vi "ball_demo.vi"() -> ()   [LabVIEW 2011]
panel:
  in  "stop":bool
  in  "Initial velocity":dbl(knob) scale=-15.0..15.0
  in  "Coefficient of Restitution":dbl(knob)=1.0 scale=0.0..1.5
  in  "Initial height":dbl(knob)=5.0 scale=5.0..20.0
  out "LabVIEW":cluster{dbl[], dbl[]}[](graph)
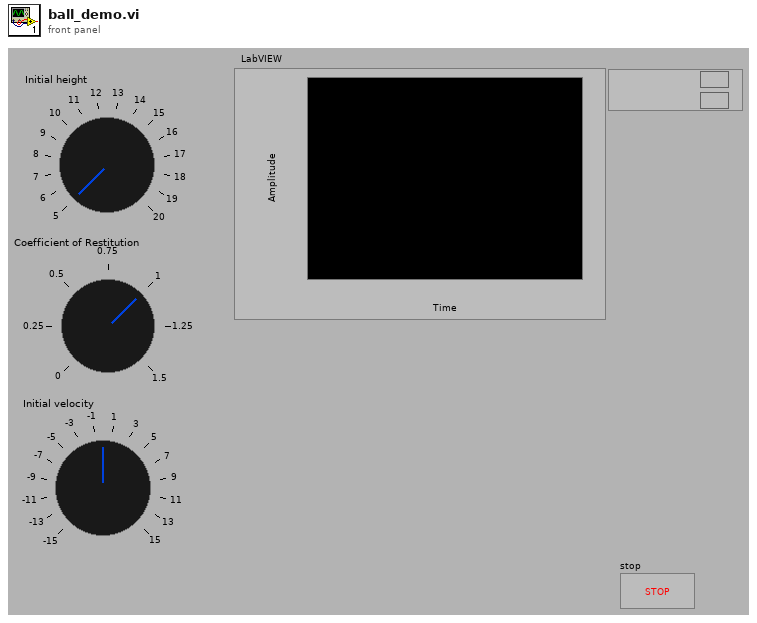
[diagram p1: front panel]
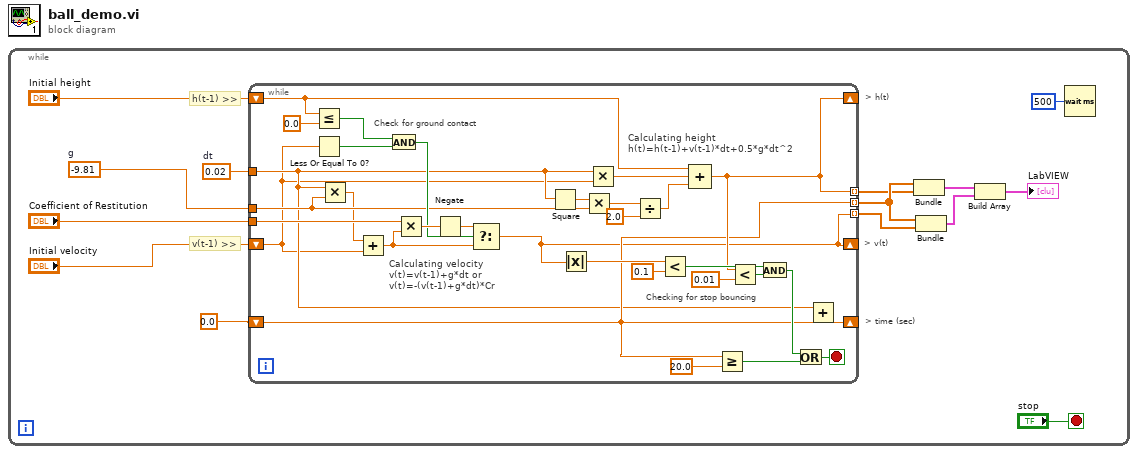
[diagram p0: block diagram]
diagram:
  n1 = while {
    stop <- "stop" stop-if-true
    w1 = 0.02  # dt
    w2 = -9.81  # g
    # "> v(t)"
    # "v(t-1) >>"
    # "h(t-1) >>"
    # "> h(t)"
    # "> time (sec)"
    n2 = while {
      tunnel: w1 -> [w19]
      tunnel: w2 -> [w27]
      shift-right: [w18] -> _
      shift-left: "Initial velocity" -> [w17]
      shift-right: [w23] -> _
      shift-left: "Initial height" -> [w38]
      tunnel: "Coefficient of Restitution" -> [w29]
      shift-right: [w21] -> _
      shift-left: 0.0 ("time") -> [w20]
      tunnel: [w23] -> w13 mode=indexing
      tunnel: [w18] -> w12 mode=indexing
      tunnel: [w20] -> w14 mode=indexing
      stop <- w34 stop-if-true
      # "Checking for stop bouncing"
      # "Calculating velocity\nv(t)=v(t-1)+g*dt or\nv(t)=-(v(t-1)+g*dt)*Cr"
      # "Check for ground contact"
      # "Calculating height\nh(t)=h(t-1)+v(t-1)*dt+0.5*g*dt^2"
      n3 = Less Or Equal?(x=w38, y=0.0) -> (x <= y?=w41:bool)
      n4 = Less Or Equal To 0?(x=w17) -> (x <= 0?=w40:bool)
      n5 = Multiply(x=w19, y=w27) -> (x*y=w16:dbl)
      n6 = Add(x=w16, y=w17) -> (x+y=w15:dbl)
      n7 = And(x=w41, y=w40) -> (x .and. y?=w39:bool)
      n8 = Multiply(x=w29, y=w15) -> (x*y=w43:dbl)
      n9 = Negate(x=w43) -> (-x=w42:dbl)
      n10 = Select(t=w42, s=w39, f=w15) -> (s? t:f=w18:dbl)
      n11 = Square(x=w19) -> (x^2=w28:dbl)
      n12 = Absolute Value(x=w18) -> (abs(x)=w36:dbl)
      n13 = Multiply(x=w28, y=w27) -> (x*y=w26:dbl)
      n14 = Multiply(x=w19, y=w17) -> (x*y=w45:dbl)
      n15 = Divide(x=w26, y=2.0) -> (x/y=w24:dbl)
      n16 = Less?(x=w36, y=0.1) -> (x < y?=w30:bool)
      n17 = Compound Arithmetic op=ADD(w38, w45, w24) -> (w23:dbl)
      n18 = Greater Or Equal?(x=w20, y=20.0 ("x")) -> (x >= y?=w33:bool)
      n19 = Less?(x=w23, y=0.01) -> (x < y?=w31:bool)
      n20 = And(x=w30, y=w31) -> (x .and. y?=w32:bool)
      n21 = Or(x=w32, y=w33) -> (x .or. y?=w34:bool)
      n22 = Add(x=w19, y=w20) -> (x+y=w21:dbl)
    }
    n23 = Bundle(w14, w13) -> (w11:cluster{dbl[], dbl[]})  [unwired: 1 in]
    n24 = Bundle(w14, w12) -> (w10:cluster{dbl[], dbl[]})  [unwired: 1 in]
    n25 = Build Array(w11, w10) -> (→"LabVIEW":cluster{dbl[], dbl[]}[])
    n26 = Wait (ms)(milliseconds to wait=u32 500) -> ()  [unwired: 1 out]
  }
